vi "Get Object Dict.vi"(11 "EDS in":refnum<class "EDS.lvclass">) -> (2 "Object Dictionary":refnum<class "Dictionary.lvclass">, 3 "EDS out":refnum<class "EDS.lvclass">)   [LabVIEW 2024, in "EDS.lvclass"]
uses:
  EDS.lvclass
  Object Dictionary/Dictionary.lvclass
  EDS.lvclass/EDS.ctl
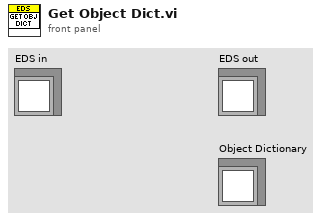
[diagram p1: front panel]
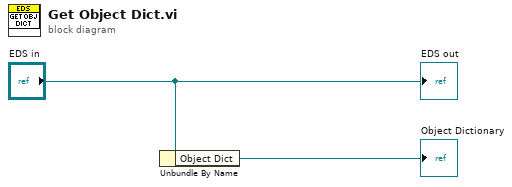
[diagram p0: block diagram]
diagram:
  n1 = Unbundle By Name("EDS in") -> ("Object Dict"=→"Object Dictionary":refnum<class "Dictionary.lvclass">)
  "EDS out" <- "EDS in"
